vi "open_python_from_text.vi"(11 "Python Function:":string) -> (0 "error out":errorcluster, 1 "function name":string, 2 "module path":path, 3 "Refnum out":refnum<k35>)   [LabVIEW 2021]
uses:
  <vilib>/regexp/Match Regular Expression.xnode
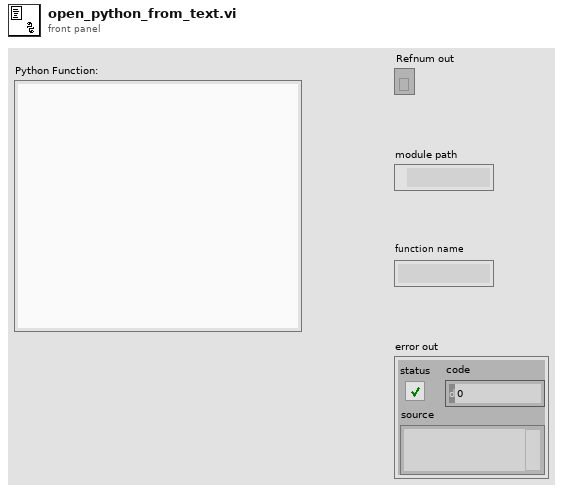
[diagram p1: front panel]
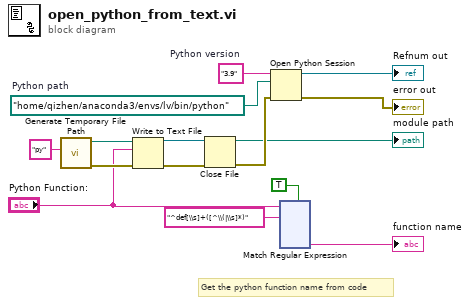
[diagram p0: block diagram]
diagram:
  w2 = path "/home/qizhen/anaconda3/envs/lv/bin/python"  # Python path
  w1 = "3.9"  # Python version
  # "Get the python function name from code"
  n1 = call <vilib>:"Generate Temporary File Path.vi"("Temporary File Extension (tmp)"="py") -> ("error out"=w13:errorcluster, "Unique Temporary File Path"=w7:path)  [unwired: 9 in]
  n2 = Write to Text File(file (use dialog)=w7, text="Python Function:", error in=w13) -> (refnum out=w8:refnum<file>, error out=w10:errorcluster)  [unwired: 1 in, 1 out]
  n3 = Close File(refnum=w8, error in=w10) -> (path=→"module path":path, error out=w14:errorcluster)
  n4 = Open Python Session(python version=w1, python path=w2, 3:w14) -> (session out=→"Refnum out":refnum<k35>, error out=→"error out":errorcluster)
  n5 = xnode "Match Regular Expression"("input string"="Python Function:", "regular expression"="^def[\\s]+([^\\(|\\s]*)", "multiline? (F)"=TRUE) -> ("submatch 1"=→"function name":string)  [unwired: 3 in, 5 out]
